vi "Sensor 2P.vi"(4 "Xmax":dbl=100.0 min=-100000.0 max=100000.0 step=0.0010000000474974513, 6 "Xmin":dbl min=-100000.0 max=100000.0 step=0.0010000000474974513, 9 "Ymin":dbl min=-100000.0 max=100000.0 step=0.0010000000474974513, 10 "Ymax":dbl=100.0 min=-100000.0 max=100000.0 step=0.0010000000474974513, 11 "X":dbl step=0.009999999776482582) -> (3 "Y":dbl format="%#.2f")   [LabVIEW 2019, in "Inputs.lvlib"]
uses:
  Inputs.lvlib
panel:
  # "(X - Xmin)\n Y= -----------*(Ymax - Ymin)+Ymin\n    (Xmax - Xmin)"
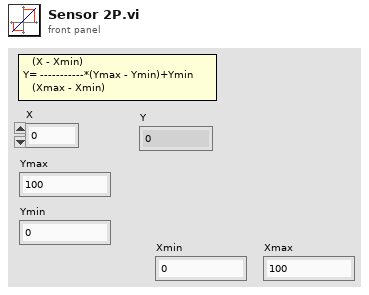
[diagram p1: front panel]
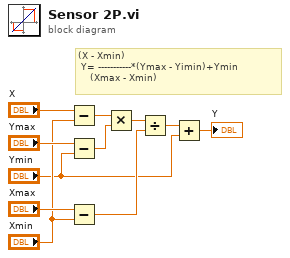
[diagram p0: block diagram]
diagram:
  # "(X - Xmin)\n Y= -----------*(Ymax - Yimin)+Ymin\n    (Xmax - Xmin)"
  n1 = Subtract(x="X", y="Xmin") -> (x-y=w9:dbl)
  n2 = Subtract(x="Ymax", y="Ymin") -> (x-y=w8:dbl)
  n3 = Subtract(x="Xmax", y="Xmin") -> (x-y=w4:dbl)
  n4 = Multiply(x=w9, y=w8) -> (x*y=w7:dbl)
  n5 = Divide(x=w7, y=w4) -> (x/y=w3:dbl)
  n6 = Add(x=w3, y="Ymin") -> (x+y=→"Y":dbl)
